vi "_Calculate Check Sum.vi"(1 "Stream":string) -> (0 "Checksum":u16)   [LabVIEW 2012]
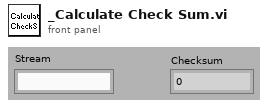
[diagram p1: front panel]
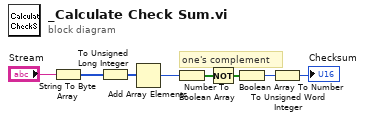
[diagram p0: block diagram]
diagram:
  # "one's complement"
  n1 = String To Byte Array(string="Stream") -> (unsigned byte array=w8:u8[])
  n2 = To Unsigned Long Integer(number=w8) -> (unsigned 32bit integer=w7:u32[])
  n3 = Add Array Elements(numeric array=w7) -> (sum=w4:u32)
  n4 = Number To Boolean Array(number=w4) -> (Boolean array=w6:bool[])
  n5 = Not(x=w6) -> (.not. x?=w5:bool[])
  n6 = Boolean Array To Number(Boolean array=w5) -> (number=w2:u32)
  n7 = To Unsigned Word Integer(number=w2) -> (unsigned 16bit integer=→"Checksum":u16)
